vi "Main FPGA 5-axis Servo.vi"() -> ()   [LabVIEW 2014]
uses:
  <vilib>/Motion/MotorControl/_s/nism.encoder.config.ctl
  <vilib>/Motion/MotorControl/_s/nism.encoder.incremental.config.ctl
  <vilib>/Motion/MotorControl/_s/nism.incremental.indexCriteria.ctl
  <vilib>/Motion/MotorControl/_s/nism.pid.gains.fxp.18.ctl
  <vilib>/Motion/MotorControl/_s/nism.pi.v.outputRange.fxp.6.12.ctl
  <vilib>/Motion/MotorControl/_s/nism.mdo.splineData.ctl
  <vilib>/Motion/MotorControl/_s/nism.splineInterpolation.type.ctl
  <vilib>/Motion/SoftMotion/Synchronization/nism.softmotionScan.timerConfig.ctl
  <vilib>/Platform/TimedLoop/XDataNode/timing_clust.ctl
  <vilib>/Platform/TimedLoop/XDataNode/nitl_modes.ctl
  <vilib>/Platform/TimedLoop/XDataNode/wakeup.ctl
  <vilib>/Motion/MotorControl/_s/nism.digitalInputs.portA.ctl
  <vilib>/rvi/Emulation/niFpgaGetClockAttributes.vi
  <vilib>/rvi/Emulation/niFpgaSctlEmulationGetInTimedLoop.vi
  <vilib>/rvi/Emulation/niFpgaEmulationReportErrorSimple.vi
  Global FPGA 5-axis.vi
  <vilib>/Motion/MotorControl/_s/nism.interpretControlRegister.indexed.vi
  <vilib>/rvi/Emulation/niFpgaProcessEmulError.vi
  <vilib>/Motion/MotorControl/_s/nism.mdo.read.encoder.vi
  <vilib>/Motion/MotorControl/_s/nism.mdo.read.positionLoopSyncData.vi
  <vilib>/Motion/MotorControl/_s/nism.mdo.read.splineData.vi
  <vilib>/Motion/MotorControl/_s/nism.generateStatusRegister.indexed.vi
  <vilib>/rvi/eio/common/nirviEmuTemplateMethod_errors.vi
  <vilib>/rvi/Emulation/niFpgaCriticalErrorInLSC.vi
  <vilib>/Motion/MotorControl/_s/nism.splineInterpolation.fxp.3.index.vi
  <vilib>/Motion/MotorControl/_s/nism.pid.simple.fxp.index.2.vi
  <vilib>/Motion/MotorControl/_s/nism.mdo.handler.indexed.vi
  <vilib>/Motion/MotorControl/_s/nism.digitalFilter.indexed.vi
  <vilib>/Motion/MotorControl/_s/nism.interpretDIOControl.portA.multiple.vi
  <vilib>/Motion/MotorControl/_s/nism.generateDIOStatus.portA.indexed.2.vi
  <vilib>/Motion/SoftMotion/Synchronization/nism.rioScan.generateSyncScan.vi
  <vilib>/Motion/MotorControl/_s/nism.incremental.p.2.vi
  <vilib>/eio/EIONode/EIONode.xnode
  <vilib>/Platform/TimedLoop/XDataNode/XDataNode.xnode
  <vilib>/Motion/MotorControl/NI_SoftMotion_MotorControlIP.lvlib
  <vilib>/Platform/TimedLoop/XDataNode/XDNodeRunTimeDep.lvlib
  <vilib>/Motion/SoftMotion/Synchronization/NI_SoftMotion_Synchronization.lvlib
  <vilib>/rvi/Analysis/measure/butterworth/XNode/niFpgaButterworthFilter.xnode
panel:
  out "Interpolated Position":fxp<+/-,64,32>[](array[numeric])
  in  "Encoder Config (Manual)":T1={"active states"={"line a active high?"=FALSE, "line b active high?"=FALSE, "index active high?"=FALSE}, "index criteria"={"a"=FALSE, "b"=FALSE, "z"=FALSE}, "vel. filter coeffs."=[0, 0, 0]} caption="encoder config"
  in  "Velocity Filter Active?":bool
  in  "Reset Encoder 5":bool caption="reset"
  in  "Reset Encoder 4":bool caption="reset"
  in  "Reset Encoder 3":bool caption="reset"
  out "position loop sync":T4
  out "spline":T5 {"spline type" items=["cubic b spline", "catmull-rom spline", "linear"]}
  in  "Reset Encoder 2":bool caption="reset"
  out "Velocity Feedback":i16[](array[numeric])
  out "pos. error":i16[](array[numeric])
  out "pos. error exceeded":bool[](array[boolean])
  in  "calls per sample (vel)":u16=2000 caption="calls per sample"
  in  "Limit Ranges":T7[](array[typedef])=[{"output low"=0.0, "output high"=0.0}, {"output low"=0.0, "output high"=0.0}, {"output low"=0.0, "output high"=0.0}, {"output low"=0.0, "output high"=0.0}, {"output low"=0.0, "output high"=0.0}]
  in  "Gains":T8[](array[typedef])=[{"kp"=0.0, "kd"=0.0, "ki"=0.0}, {"kp"=0.0, "kd"=0.0, "ki"=0.0}, {"kp"=0.0, "kd"=0.0, "ki"=0.0}, {"kp"=0.0, "kd"=0.0, "ki"=0.0}, {"kp"=0.0, "kd"=0.0, "ki"=0.0}]
  out "AO Check":fxp<+/-,20,5>[](array[numeric])
  in  "AO Manual":fxp<+/-,20,5>[](array[numeric])=[0.0, 0.0, 0.0, 0.0, 0.0]
  out "Position Feedback":i32[](array[numeric])
  in  "Reset Encoder 1":bool caption="reset"
  out "corrected period":u16
  in  "AO Disabled?":bool
  out "PID loop time (ticks)":u32
  in  "AO Override?":bool
  in  "position error limit":i16=10000
  in  "Encoder filter value (us) Manual":u16=10
  out "encoder config":T1
  out "Home Limits":bool[](array[boolean])
  out "Fwd Limits":bool[](array[boolean])
  out "Rev Limits":bool[](array[boolean])
  out "Drive Enable":bool[](array[boolean])
  in  "Enable value":bool
  in  "Drive Enable override?":bool
  in  "Sync Value":bool
  in  "Sync Enable override?":bool
  out "Sync is Fault":bool
  out "Sync is Locked":bool
  # "Synchronization Loop"
  # "Control Status Loop"
  # "Notes: \n1. This VI provides the communication interface between the NI SoftMotion Engine and the LabVIEW FPGA Module. You must compile this VI for a specific FPGA target before use. After compiling, run the VI before running any of the Express VI examples. For information on moving this example to another FPGA target, refer to ni.com/info and enter info code fpgaex.\n\n2. Only use the Reset Axis button if you are unable to communicate with the axis by any other means. This button resets the device state machine and other VIs to a known state. After resetting the axis, switch the NI Scan Engine from Active Mode to Configuration Mode, then back to Active Mode, before attempting to enable the axis."
  # "(These two buttons \nare for testing\npurposes.)"
  # "(These two buttons \nare for testing\npurposes.)"
  # "Position/PID Loop"
  # "Parameter Check"
  # "AO Debug"
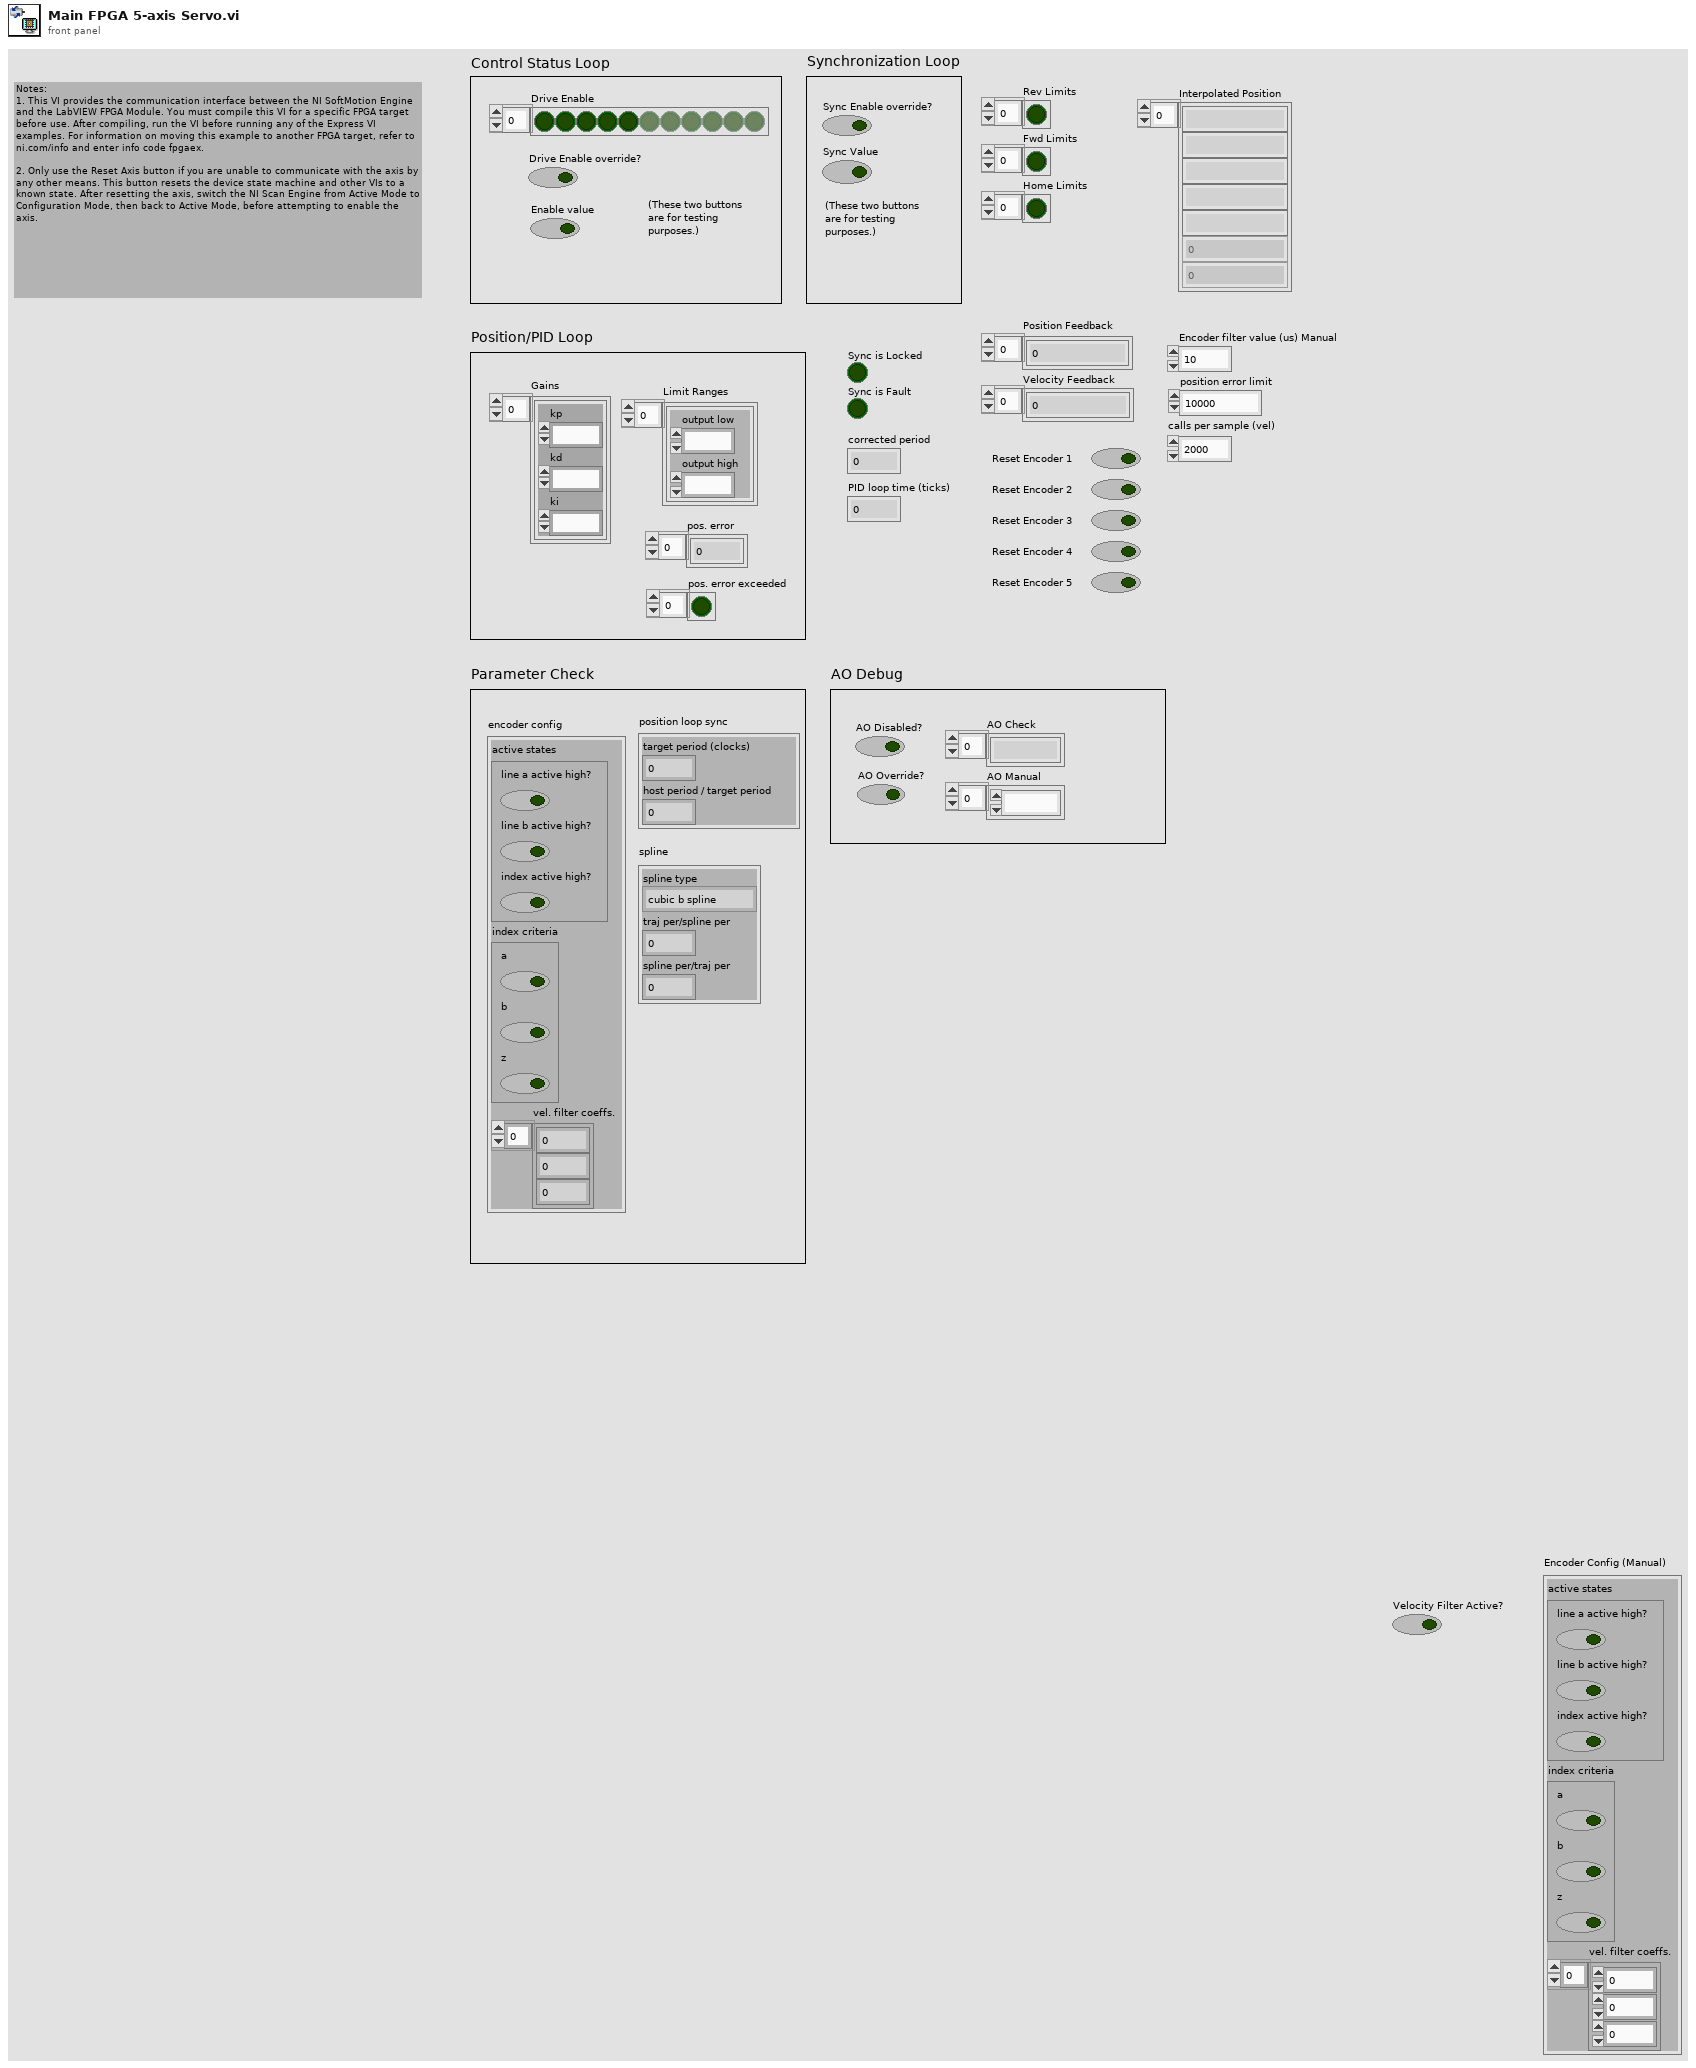
[diagram p1: front panel]
types:
  T1 = typedef "NI_SoftMotion_MotorControlIP.lvlib/nism.encoder.config.ctl" = cluster{"active states":T2, "index criteria":T3, "vel. filter coeffs.":i32[]}
  T2 = typedef "NI_SoftMotion_MotorControlIP.lvlib/nism.encoder.incremental.config.ctl" = cluster{"line a active high?":bool, "line b active high?":bool, "index active high?":bool}
  T3 = typedef "NI_SoftMotion_MotorControlIP.lvlib/nism.incremental.indexCriteria.ctl" = cluster{"a":bool, "b":bool, "z":bool}
  T4 = typedef "NI_SoftMotion_Synchronization.lvlib/nism.softmotionScan.timerConfig.ctl" = cluster{"target period (clocks)":u16, "host period / target period":u16}
  T5 = typedef "NI_SoftMotion_MotorControlIP.lvlib/nism.mdo.splineData.ctl" = cluster{"spline type":T6, "traj per/spline per":u16, "spline per/traj per":fxp<+,32,0>}
  T6 = typedef "NI_SoftMotion_MotorControlIP.lvlib/nism.splineInterpolation.type.ctl" = u16
  T7 = typedef "NI_SoftMotion_MotorControlIP.lvlib/nism.pi.v.outputRange.fxp.6.12.ctl" = cluster{"output low":fxp<+/-,18,6>, "output high":fxp<+/-,18,6>}
  T8 = typedef "NI_SoftMotion_MotorControlIP.lvlib/nism.pid.gains.fxp.18.ctl" = cluster{"kp":fxp<+,18,7>, "kd":fxp<+,18,7>, "ki":fxp<+,18,0>}
  T9 = typedef "XDNodeRunTimeDep.lvlib/timing_clust.ctl" = cluster{"Expected End [f-1]":u64, "Actual End [f-1]":u64, "Finished Late? [f-1]":bool, "Expected End [i-1]":u64, "Actual End [i-1]":u64, "Finished Late? [i-1]":bool, "Expected Start [i]":u64, "Actual Start [i]":u64, "Expected Start [f]":u64, "Actual Start [f]":u64, "Source Name":string, "Structure Name":string, "Period":i64, "Deadline":i64, "Offset":i64, "Start":i64, "Priority":i32, "Timeout":i32, "Mode":T10, "Wakeup Reason":T11, "Error":errorcluster, "Source Type":string, "Secondary Source Type":string, "Global End Time":u64, "Global Start Time":u64, "Frame Duration":u64, "Iteration Duration":u64, "Assigned CPU":i32, "I/O Scan Engine Mode":u32}
  T10 = typedef "XDNodeRunTimeDep.lvlib/nitl_modes.ctl" = enum32{"No Change", "Process missed periods, maintain original phase", "Discard missed periods, maintain original phase", "Process missed periods, ignore original phase", "Discard missed periods, ignore original phase"}
  T11 = typedef "XDNodeRunTimeDep.lvlib/wakeup.ctl" = enum32{"Normal", "Aborted", "Asynchronous wakeup", "Timing source error", "Timed loop error", "Timeout"}
  T12 = typedef "NI_SoftMotion_MotorControlIP.lvlib/nism.digitalInputs.portA.ctl" = cluster{"reverse limit":bool, "forward limit":bool, "home switch":bool, "digital input 0":bool, "digital input 1":bool, "digital input 2":bool, "digital input 3":bool}
  T13 = typedef "NI_SoftMotion_MotorControlIP.lvlib/nism.dio.portA.config.2.ctl" = cluster{"digital filter (us)":u16[], "safe state":T14[]}
  T14 = typedef "nism.safeStates.ctl" = enum8{"Low", "High", "No Change"}
  T15 = typedef "NI_SoftMotion_Synchronization.lvlib/nism.softmotionScan.timerControl.ctl" = cluster{"sm scan":bool, "sm scan count":u32, "sm scan enabled":bool}
  T16 = typedef "NI_SoftMotion_MotorControlIP.lvlib/nism.interpretControlRegister.stateTransition.ctl" = enum8{"Invalid", "Start --> Initializing", "Initializing --> Disabled", "Disabled --> Ready To Switch On", "Ready To Switch On --> Switched On", "Ready To Switch On --> Disable", "Switched On --> Operation Enable", "Switched On --> Ready To Switch On", "Switched On --> Disabled", "Operation Enable --> Switched On", "Operation Enable --> Ready To Switch On", "Operation Enable --> Disabled", "Fault --> Disabled", "Any --> Fault", "None"}
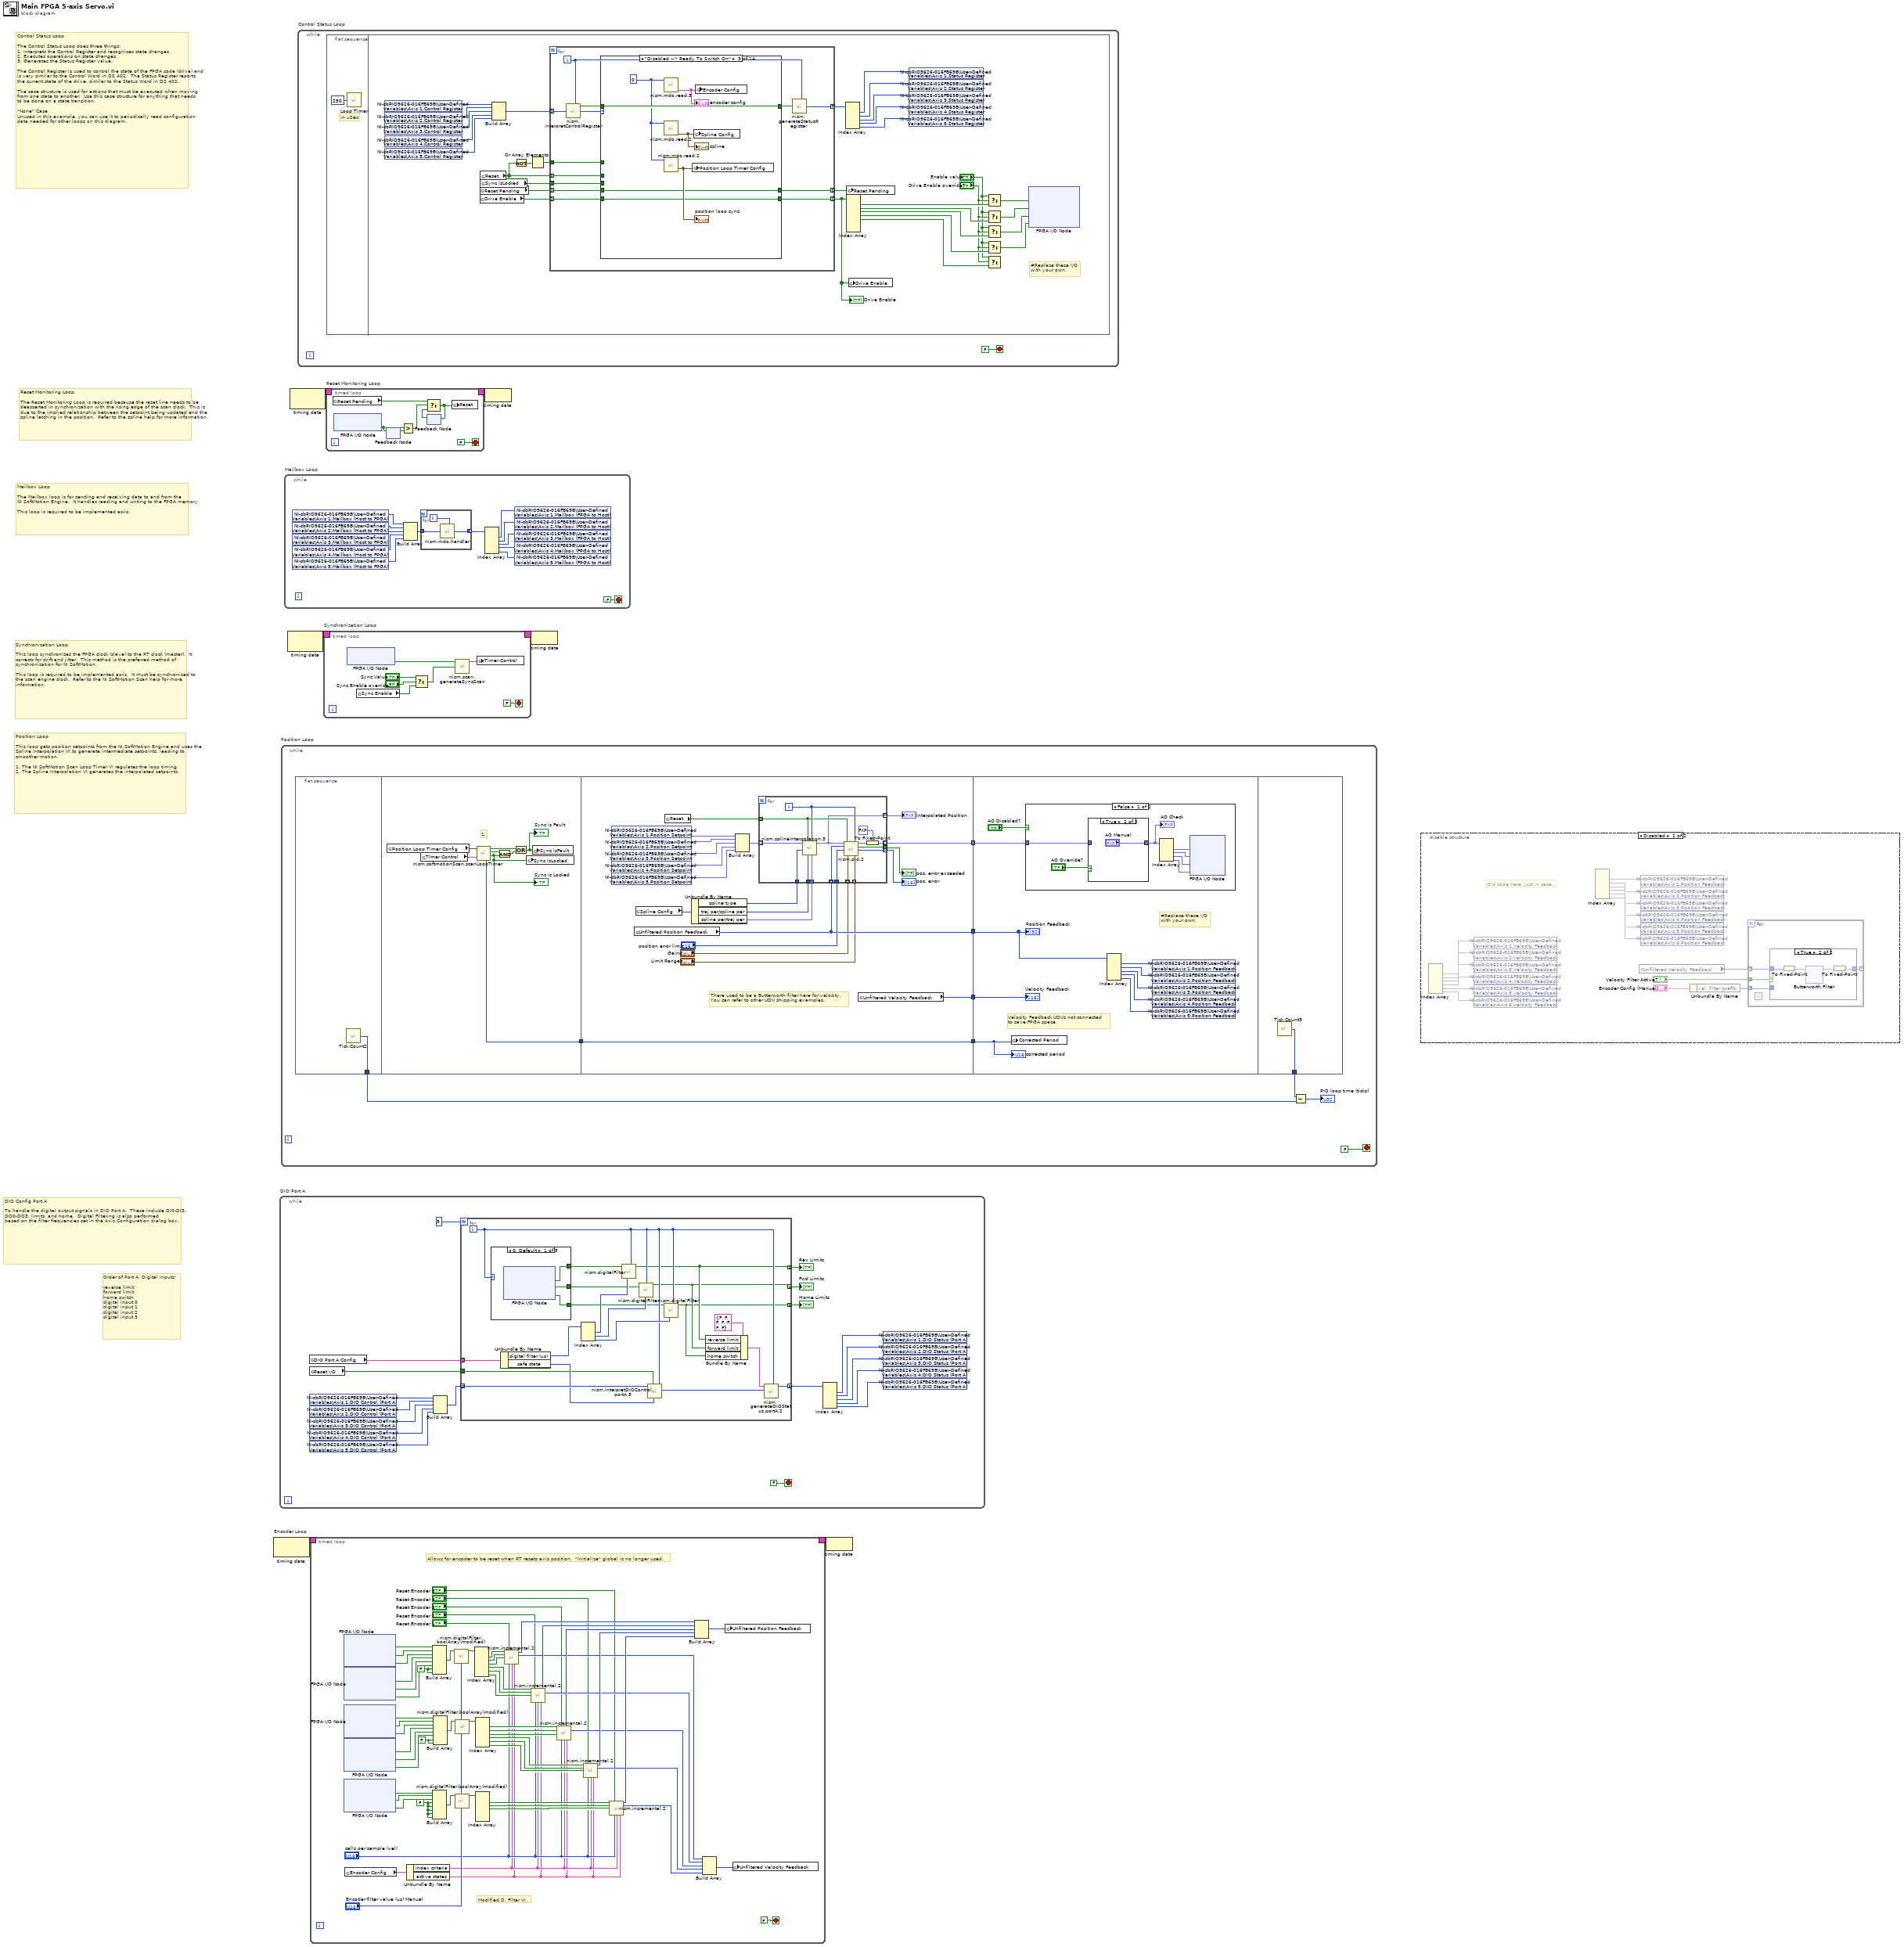
[diagram p0: block diagram]
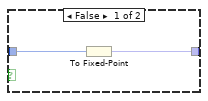
[diagram p2: hidden frame]
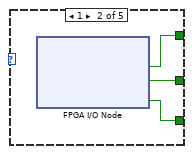
[diagram p4: hidden frame]
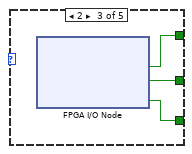
[diagram p5: hidden frame]
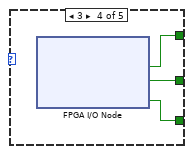
[diagram p6: hidden frame]
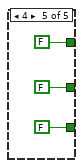
[diagram p7: hidden frame]
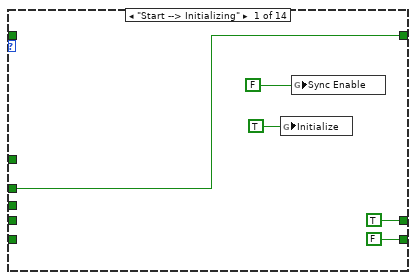
[diagram p10: hidden frame]
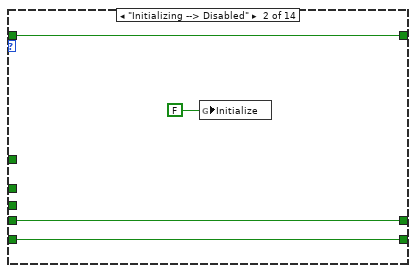
[diagram p11: hidden frame]
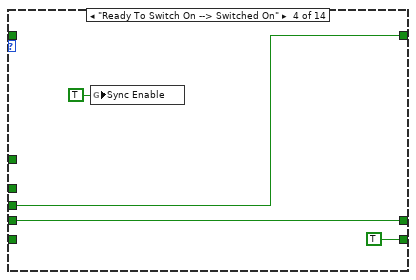
[diagram p12: hidden frame]
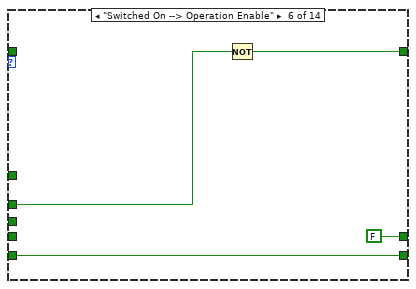
[diagram p14: hidden frame]
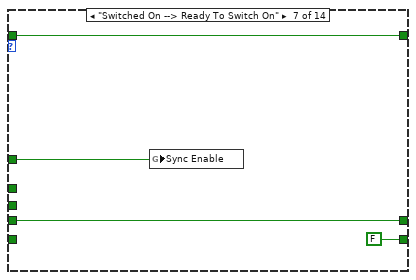
[diagram p15: hidden frame]
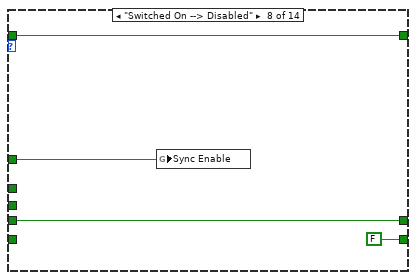
[diagram p16: hidden frame]
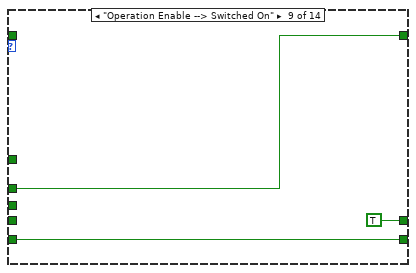
[diagram p17: hidden frame]
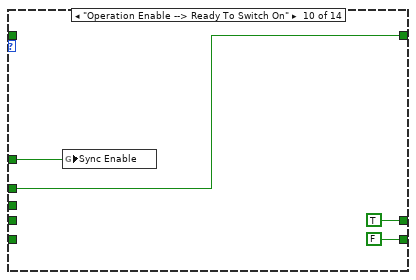
[diagram p18: hidden frame]
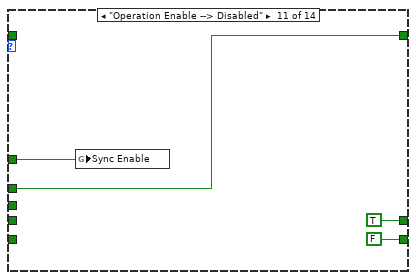
[diagram p19: hidden frame]
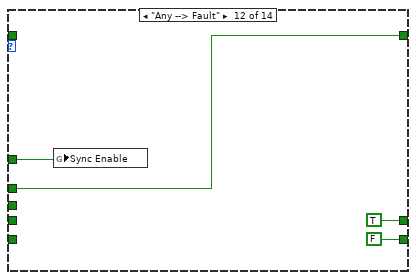
[diagram p20: hidden frame]
diagram:
  # "DIO Config Port A\n\nTo handle the digital output signals in DIO Port A.  These include DI0-DI3, DO0-DO3, limits, and home.  Digital Filtering is also performed\nbased on the filter frequencies set in the Axis Configuration dialog box."
  # "Order of Port A, Digital Inputs:\n\nreverse limit\nforward limit\nhome switch\ndigital input 0\ndigital input 1\ndigital input 2\ndigital input 3"
  # "Position Loop\n\nThis loop gets position setpoints from the NI SoftMotion Engine and uses the Spline Interpolation VI to generate intermediate setpoints, leading to smoother motion.\n\n1. The NI SoftMotion Scan Loop Timer VI regulates the loop timing. \n2. The Spline Interpolation VI generates the interpolated setpoints."
  # "Synchronization Loop\n\nThis loop synchronizes the FPGA clock (slave) to the RT clock (master).  It corrects for drift and jitter.  This method is the preferred method of synchronization for NI SoftMotion.\n\nThis loop is required to be implemented as-is.  It must be synchronized to the scan engine clock.  Refer to the NI SoftMotion Scan help for more information."
  # "Mailbox Loop\n\nThe Mailbox loop is for sending and receiving data to and from the \nNI SoftMotion Engine.  It handles reading and writing to the FPGA memory.\n\nThis loop is required to be implemented as-is."
  # "Reset Monitoring Loop\n\nThe Reset Monitoring Loop is required because the reset line needs to be deasserted in synchronization with the rising edge of the scan clock.  This is due to the implied relationship between the setpoint being updated and the spline latching in the position.  Refer to the spline help for more information."
  # "Control Status Loop\n\nThe Control Status Loop does three things:\n1. Interprets the Control Register and recognizes state changes.\n2. Executes operations on state changes.\n3. Generates the Status Register value.\n\nThe Control Register is used to control the state of the FPGA code (drive) and is very similar to the Control Word in DS 402.  The Status Register reports the current state of the drive, similar to the Status Word in DS 402.\n\nThe case structure is used for actions that must be executed when moving from one state to another.  Use this case structure for anything that needs to be done on a state transition.\n\n\"None\" Case\nUnused in this example, you can use it to periodically read configuration data needed for other loops on this diagram."
  n1 = node-c288() -> (w2:T9)  [unwired: 1 in]
  n2 = while "DIO Port A" {
    stop <- FALSE stop-if-true
    n3 = global read "Global FPGA 5-axis.vi" "DIO Port A Config"() -> (w24:T13)
    n4 = global read "Global FPGA 5-axis.vi" "Reset I/O"() -> (w23:bool)
    n5 = shared-variable "NI-sbRIO9626-016FB69B\\User-Defined Variables\\Axis 1.DIO Control (Port A)"() -> (w21:u32)  [unwired: 1 in, 1 out]
    n6 = shared-variable "NI-sbRIO9626-016FB69B\\User-Defined Variables\\Axis 2.DIO Control (Port A)"() -> (w20:u32)  [unwired: 1 in, 1 out]
    n7 = shared-variable "NI-sbRIO9626-016FB69B\\User-Defined Variables\\Axis 3.DIO Control (Port A)"() -> (w19:u32)  [unwired: 1 in, 1 out]
    n8 = shared-variable "NI-sbRIO9626-016FB69B\\User-Defined Variables\\Axis 4.DIO Control (Port A)"() -> (w18:u32)  [unwired: 1 in, 1 out]
    n9 = shared-variable "NI-sbRIO9626-016FB69B\\User-Defined Variables\\Axis 5.DIO Control (Port A)"() -> (w17:u32)  [unwired: 1 in, 1 out]
    n10 = Build Array(w21, w20, w19, w18, w17) -> (w16:u32[])
    n11 = for {
      N: 5 -> [_]
      tunnel: [w43] -> w10 mode=indexing
      tunnel: w16 -> [w42] mode=indexing
      tunnel: w24 -> [w39]
      tunnel: w23 -> [w37]
      tunnel: [w28] -> w9 mode=indexing
      tunnel: [w27] -> w8 mode=indexing
      tunnel: [w26] -> w7 mode=indexing
      i -> [w32]
      n12 = case shown="0, Default" w32 {
        tunnel: [w47 w50 w53 w56 FALSE ("RMC/DIO44")] -> w31
        tunnel: [w45 w48 w51 w54 FALSE ("RMC/DIO61")] -> w30
        tunnel: [w46 w49 w52 w55 FALSE ("RMC/DIO77")] -> w29
        frame 0, Default {
          n13 = xnode "FPGA I/O Node"() -> ("RMC/DIO29"=w47:bool, "RMC/DIO93"=w46:bool, "RMC/DIO11"=w45:bool)  [unwired: 3 in, 3 out]
        }
        frame 1 {
          n14 = xnode "FPGA I/O Node"() -> ("RMC/DIO44"=w50:bool, "RMC/DIO77"=w49:bool, "RMC/DIO61"=w48:bool)  [unwired: 3 in, 3 out]
        }
        frame 2 {
          n15 = xnode "FPGA I/O Node"() -> ("RMC/DIO31"=w53:bool, "RMC/DIO95"=w52:bool, "RMC/DIO13"=w51:bool)  [unwired: 3 in, 3 out]
        }
        frame 3 {
          n16 = xnode "FPGA I/O Node"() -> ("RMC/DIO47"=w56:bool, "RMC/DIO46"=w55:bool, "RMC/DIO79"=w54:bool)  [unwired: 3 in, 3 out]
        }
        frame 4 {
        }
      }
      n17 = Unbundle By Name(w39) -> ("digital filter (us)"=w33:u16[], "safe state"=w38:T14[])
      n18 = Index Array(array=w33) -> (element #1=w34:u16, element #2=w35:u16, element #3=w36:u16)  [unwired: 3 in]
      n19 = call-poly <vilib>:"nism.digitalFilter.vi"("index"=w32, "filter value (us)"=w34, "input signal"=w31) -> ("output signal"=w28:bool)  [unwired: 8 in]
      n20 = call-poly <vilib>:"nism.digitalFilter.vi"("index"=w32, "filter value (us)"=w35, "input signal"=w29) -> ("output signal"=w27:bool)  [unwired: 8 in]
      n21 = call-poly <vilib>:"nism.interpretDIOControl.portA.3.vi"("index"=w32, "safe state"=w38, "reset"=w37, "dio control(port a)"=w42) -> ("reset latches"=w44:u8)  [unwired: 6 in, 1 out]
      n22 = call-poly <vilib>:"nism.digitalFilter.vi"("index"=w32, "filter value (us)"=w36, "input signal"=w30) -> ("output signal"=w26:bool)  [unwired: 8 in]
      n23 = Bundle By Name(cluster=T12 {"reverse limit"=FALSE, "forward limit"=FALSE, "home switch"=FALSE, "digital input 0"=FALSE, "digital input 1"=FALSE, "digital input 2"=FALSE, "digital input 3"=FALSE} ("$(driveInterface.digitalInputs.shortName)"), "reverse limit"=w28, "forward limit"=w27, "home switch"=w26) -> (w40:T12)
      n24 = call-poly <vilib>:"nism.generateDIOStatus.portA.2.vi"("index"=w32, "reset latches"=w44, "digital inputs"=w40) -> ("dio status(port a)"=w43:u32)  [unwired: 8 in]
    }
    "Rev Limits" <- w9
    "Fwd Limits" <- w8
    "Home Limits" <- w7
    n25 = Index Array(array=w10) -> (element #1=w15:u32, element #2=w14:u32, element #3=w13:u32, element #4=w12:u32, element #5=w11:u32)  [unwired: 5 in]
    n26 = shared-variable "NI-sbRIO9626-016FB69B\\User-Defined Variables\\Axis 1.DIO Status (Port A)"(w15) -> ()  [unwired: 1 in, 1 out]
    n27 = shared-variable "NI-sbRIO9626-016FB69B\\User-Defined Variables\\Axis 2.DIO Status (Port A)"(w14) -> ()  [unwired: 1 in, 1 out]
    n28 = shared-variable "NI-sbRIO9626-016FB69B\\User-Defined Variables\\Axis 3.DIO Status (Port A)"(w13) -> ()  [unwired: 1 in, 1 out]
    n29 = shared-variable "NI-sbRIO9626-016FB69B\\User-Defined Variables\\Axis 4.DIO Status (Port A)"(w12) -> ()  [unwired: 1 in, 1 out]
    n30 = shared-variable "NI-sbRIO9626-016FB69B\\User-Defined Variables\\Axis 5.DIO Status (Port A)"(w11) -> ()  [unwired: 1 in, 1 out]
  }
  n31 = while "Position Loop" {
    stop <- FALSE stop-if-true
    n32 = flat-sequence {
      tunnel: [w69] -> w63
      tunnel: [w70] -> w66
      tunnel: [w94] -> w67
      tunnel: w66 -> [w94]
      tunnel: [w84] -> w65
      tunnel: [w88] -> w61
      tunnel: [w79] -> w60
      tunnel: w67 -> [w124]
      tunnel: w65 -> [w115]
      tunnel: w61 -> [w123]
      tunnel: w60 -> [w121]
      tunnel: [w134] -> w64
      frame #0 {
        n33 = call "Tick Count2"() -> ("Tick Count(Ticks)"=w69:u32)
      }
      frame #1 {
        # "1."
        n34 = global read "Global FPGA 5-axis.vi" "Position Loop Timer Config"() -> (w72:T4)
        n35 = global read "Global FPGA 5-axis.vi" "Timer Control"() -> (w71:T15)
        n36 = call <vilib>:"nism.softmotionScan.scanLoopTimer.vi"("timer control"=w71, "timer config"=w72) -> ("scan running?"=w74:bool, "finished late?"=w76:bool, "fault occurred?"=w77:bool, "corrected period"=w70:u16)  [unwired: 5 in, 1 out]
        "Sync is Locked" <- w74
        n37 = Compound Arithmetic op=AND(w76, w74) -> (w75:bool)
        n38 = Compound Arithmetic op=OR(w77, w75) -> (w73:bool)
        "Sync is Fault" <- w73
        n39 = global write "Global FPGA 5-axis.vi" "Sync isLocked"(w74) -> ()
        n40 = global write "Global FPGA 5-axis.vi" "Sync isFault"(w73) -> ()
      }
      frame #2 {
        # "There used to be a Butterworth filter here for velocity.  \nYou can refer to other UDV shipping examples."
        n41 = shared-variable "NI-sbRIO9626-016FB69B\\User-Defined Variables\\Axis 1.Position Setpoint"() -> (w89:fxp<+/-,64,32>)  [unwired: 1 in, 1 out]
        n42 = shared-variable "NI-sbRIO9626-016FB69B\\User-Defined Variables\\Axis 2.Position Setpoint"() -> (w93:fxp<+/-,64,32>)  [unwired: 1 in, 1 out]
        n43 = shared-variable "NI-sbRIO9626-016FB69B\\User-Defined Variables\\Axis 3.Position Setpoint"() -> (w92:fxp<+/-,64,32>)  [unwired: 1 in, 1 out]
        n44 = shared-variable "NI-sbRIO9626-016FB69B\\User-Defined Variables\\Axis 4.Position Setpoint"() -> (w91:fxp<+/-,64,32>)  [unwired: 1 in, 1 out]
        n45 = shared-variable "NI-sbRIO9626-016FB69B\\User-Defined Variables\\Axis 5.Position Setpoint"() -> (w90:fxp<+/-,64,32>)  [unwired: 1 in, 1 out]
        n46 = global read "Global FPGA 5-axis.vi" "Unfiltered Position Feedback"() -> (w84:i32[])
        n47 = global read "Global FPGA 5-axis.vi" "Spline Config"() -> (w95:T5)
        n48 = global read "Global FPGA 5-axis.vi" "Reset"() -> (w86:bool[])
        n49 = Unbundle By Name(w95) -> ("spline type"=w98:T6, "traj per/spline per"=w97:u16, "spline per/traj per"=w96:fxp<+,32,0>)
        n50 = Build Array(w89, w93, w92, w91, w90) -> (w87:fxp<+/-,64,32>[])
        n51 = for {
          tunnel: w98 -> [w114]
          tunnel: w97 -> [w113]
          tunnel: w96 -> [w112]
          tunnel: "Limit Ranges" -> [w111] mode=indexing
          tunnel: [w101] -> w88 mode=indexing
          tunnel: w87 -> [w110] mode=indexing
          tunnel: w86 -> [w108] mode=indexing
          tunnel: w84 -> [w107] mode=indexing
          tunnel: "position error limit" -> [w106]
          tunnel: [w105] -> w81 mode=indexing
          tunnel: [w104] -> w80 mode=indexing
          tunnel: "Gains" -> [w100] mode=indexing
          tunnel: [w99] -> w78 mode=indexing
          i -> [w109]
          n52 = call-poly <vilib>:"nism.splineInterpolation.3.vi"("1 / calls per sample"=w112, "index"=w109, "calls per sample"=w113, "reset"=w108, "spline type"=w114, "x"=w110) -> ("xi"=w99:fxp<+/-,64,32>)  [unwired: 4 in, 1 out]
          n53 = call-poly <vilib>:"nism.pid.2.vi"("position setpoint"=w99, "position feedback"=w107, "position error limit"=w106, "reset"=w108, "gains"=w100, "index"=w109, "output range"=w111) -> ("current setpoint"=w102:fxp<+/-,18,6>, "pos. error exceeded"=w105:bool, "position error"=w104:i16)  [unwired: 10 in]
          n54 = To Fixed-Point(fixed-point type=fxp<+/-,20,5> 0.0 ("AO 1"), number=w102) -> (fixed-point=w101:fxp<+/-,20,5>)
        }
        "pos. error exceeded" <- w81
        "pos. error" <- w80
        "Interpolated Position" <- w78
        n55 = global read "Global FPGA 5-axis.vi" "Unfiltered Velocity Feedback"() -> (w79:i16[])
      }
      frame #3 {
        # "Velocity Feedback UDVs not connected\nto save FPGA space."
        # "#Replace these I/O\nwith your own."
        n56 = global write "Global FPGA 5-axis.vi" "Corrected Period"(w124) -> ()
        n57 = case shown="False" "AO Disabled?" {
          tunnel: w123 -> [w130 _]
          frame False {
            n58 = case shown="True" "AO Override?" {
              tunnel: w130 -> [w132 _]
              tunnel: [w132 "AO Manual"] -> w129
              frame False {
              }
              frame True {
              }
            }
            "AO Check" <- w129
            n59 = Index Array(array=w129) -> (element #1=w128:fxp<+/-,20,5>, element #2=w127:fxp<+/-,20,5>, element #3=w126:fxp<+/-,20,5>, element #4=w125:fxp<+/-,20,5>)  [unwired: 4 in]
            n60 = xnode "FPGA I/O Node"("AO0"=w128, "AO1"=w127, "AO2"=w126, "AO3"=w125) -> ()  [unwired: 4 in, 4 out]
          }
          frame True {
          }
        }
        n61 = Index Array(array=w115) -> (element #1=w120:i32, element #2=w119:i32, element #3=w118:i32, element #4=w117:i32, element #5=w116:i32)  [unwired: 5 in]
        n62 = shared-variable "NI-sbRIO9626-016FB69B\\User-Defined Variables\\Axis 1.Position Feedback"(w120) -> ()  [unwired: 1 in, 1 out]
        n63 = shared-variable "NI-sbRIO9626-016FB69B\\User-Defined Variables\\Axis 2.Position Feedback"(w119) -> ()  [unwired: 1 in, 1 out]
        n64 = shared-variable "NI-sbRIO9626-016FB69B\\User-Defined Variables\\Axis 3.Position Feedback"(w118) -> ()  [unwired: 1 in, 1 out]
        n65 = shared-variable "NI-sbRIO9626-016FB69B\\User-Defined Variables\\Axis 4.Position Feedback"(w117) -> ()  [unwired: 1 in, 1 out]
        n66 = shared-variable "NI-sbRIO9626-016FB69B\\User-Defined Variables\\Axis 5.Position Feedback"(w116) -> ()  [unwired: 1 in, 1 out]
        "corrected period" <- w124
        "Position Feedback" <- w115
        "Velocity Feedback" <- w121
      }
      frame #4 {
        n67 = call "Tick Count3"() -> ("Tick Count(Ticks)"=w134:u32)
      }
    }
    n68 = Subtract(x=w64, y=w63) -> (x-y=→"PID loop time (ticks)":u32)
  }
  n69 = while "Mailbox Loop" {
    stop <- FALSE stop-if-true
    n70 = shared-variable "NI-sbRIO9626-016FB69B\\User-Defined Variables\\Axis 1.Mailbox (Host to FPGA)"() -> (w144:u64)  [unwired: 1 in, 1 out]
    n71 = shared-variable "NI-sbRIO9626-016FB69B\\User-Defined Variables\\Axis 2.Mailbox (Host to FPGA)"() -> (w143:u64)  [unwired: 1 in, 1 out]
    n72 = shared-variable "NI-sbRIO9626-016FB69B\\User-Defined Variables\\Axis 3.Mailbox (Host to FPGA)"() -> (w142:u64)  [unwired: 1 in, 1 out]
    n73 = shared-variable "NI-sbRIO9626-016FB69B\\User-Defined Variables\\Axis 4.Mailbox (Host to FPGA)"() -> (w141:u64)  [unwired: 1 in, 1 out]
    n74 = shared-variable "NI-sbRIO9626-016FB69B\\User-Defined Variables\\Axis 5.Mailbox (Host to FPGA)"() -> (w140:u64)  [unwired: 1 in, 1 out]
    n75 = Build Array(w144, w143, w142, w141, w140) -> (w146:u64[])
    n76 = for {
      tunnel: w146 -> [w150] mode=indexing
      tunnel: [w149] -> w145 mode=indexing
      i -> [w148]
      n77 = call-poly <vilib>:"nism.mdo.handler.vi"("mbox (host to fpga)"=w150, "axis index"=w148) -> ("mbox (fpga to host)"=w149:u64)  [unwired: 7 in]
    }
    n78 = Index Array(array=w145) -> (element #1=w139:u64, element #2=w138:u64, element #3=w137:u64, element #4=w136:u64, element #5=w135:u64)  [unwired: 5 in]
    n79 = shared-variable "NI-sbRIO9626-016FB69B\\User-Defined Variables\\Axis 1.Mailbox (FPGA to Host)"(w139) -> ()  [unwired: 1 in, 1 out]
    n80 = shared-variable "NI-sbRIO9626-016FB69B\\User-Defined Variables\\Axis 2.Mailbox (FPGA to Host)"(w138) -> ()  [unwired: 1 in, 1 out]
    n81 = shared-variable "NI-sbRIO9626-016FB69B\\User-Defined Variables\\Axis 3.Mailbox (FPGA to Host)"(w137) -> ()  [unwired: 1 in, 1 out]
    n82 = shared-variable "NI-sbRIO9626-016FB69B\\User-Defined Variables\\Axis 4.Mailbox (FPGA to Host)"(w136) -> ()  [unwired: 1 in, 1 out]
    n83 = shared-variable "NI-sbRIO9626-016FB69B\\User-Defined Variables\\Axis 5.Mailbox (FPGA to Host)"(w135) -> ()  [unwired: 1 in, 1 out]
  }
  n84 = node-c288() -> (w6:T9)  [unwired: 1 in]
  n85 = node-c288() -> (w4:T9)  [unwired: 1 in]
  n86 = while "Control Status Loop" {
    stop <- FALSE stop-if-true
    n87 = flat-sequence {
      frame #0 {
        # "in uSec"
        n88 = call "Loop Timer"("Count(uSec)"=u32 250) -> ()  [unwired: 1 out]
      }
      frame #1 {
        # "#Replace these I/O\nwith your own."
        n89 = shared-variable "NI-sbRIO9626-016FB69B\\User-Defined Variables\\Axis 1.Control Register"() -> (w173:u32)  [unwired: 1 in, 1 out]
        n90 = shared-variable "NI-sbRIO9626-016FB69B\\User-Defined Variables\\Axis 2.Control Register"() -> (w172:u32)  [unwired: 1 in, 1 out]
        n91 = shared-variable "NI-sbRIO9626-016FB69B\\User-Defined Variables\\Axis 3.Control Register"() -> (w171:u32)  [unwired: 1 in, 1 out]
        n92 = shared-variable "NI-sbRIO9626-016FB69B\\User-Defined Variables\\Axis 4.Control Register"() -> (w170:u32)  [unwired: 1 in, 1 out]
        n93 = shared-variable "NI-sbRIO9626-016FB69B\\User-Defined Variables\\Axis 5.Control Register"() -> (w169:u32)  [unwired: 1 in, 1 out]
        n94 = global read "Global FPGA 5-axis.vi" "Reset Pending"() -> (w177:bool[])
        n95 = global read "Global FPGA 5-axis.vi" "Drive Enable"() -> (w176:bool[])
        n96 = global read "Global FPGA 5-axis.vi" "Reset"() -> (w178:bool[])
        n97 = global read "Global FPGA 5-axis.vi" "Sync isLocked"() -> (w183:bool)
        n98 = Build Array(w173, w172, w171, w170, w169) -> (w182:u32[])
        n99 = Not(x=w178) -> (.not. x?=w180:bool[])
        n100 = Or Array Elements(Boolean array=w180) -> (logical OR=w179:bool)
        n101 = for {
          tunnel: w178 -> [w192] mode=indexing
          tunnel: w183 -> [w191]
          tunnel: w182 -> [w193] mode=indexing
          tunnel: [w190] -> w174 mode=indexing
          tunnel: [w189] -> w181 mode=indexing
          tunnel: [w188] -> w175 mode=indexing
          tunnel: w179 -> [w187]
          tunnel: w177 -> [w186] mode=indexing
          tunnel: w176 -> [w185] mode=indexing
          i -> [w194]
          n102 = call-poly <vilib>:"nism.interpretControlRegister.vi"("control register"=w193, "axis index"=w194) -> ("transition occurred"=w195:bool, "state transition"=w184:T16)  [unwired: 6 in]
          n103 = case shown="\"Disabled --> Ready To Switch On\"" w184 {
            tunnel: w195 -> [_ w205 w212 _ w219 _ w227 w231 _ _ _ _ w251 _]
            tunnel: [w201 w205 w212 w214 w219 w223 w227 w231 w233 w236 w240 w244 w250 _] -> w196
            tunnel: w192 -> [w201 _ _ _ _ w222 _ _ w233 w236 w240 w244 _ _]
            tunnel: w191 -> [_ _ _ w214 _ _ _ _ _ _ _ _ _ _]
            tunnel: [TRUE ("Write.Reset Pending") w204 w209 w213 w218 FALSE ("Write.Reset Pending") w224 w228 TRUE ("Write.Reset Pending") TRUE ("Write.Reset Pending") TRUE ("Write.Reset Pending") TRUE ("Write.Reset Pending") w248 w253] -> w189
            tunnel: [FALSE ("Write.Drive Enable") w203 w208 TRUE ("Write.Drive Enable") w217 w220 FALSE ("Write.Drive Enable") FALSE ("Write.Drive Enable") w232 FALSE ("Write.Drive Enable") FALSE ("Write.Drive Enable") FALSE ("Write.Drive Enable") w247 w252] -> w188
            tunnel: w187 -> [_ _ _ _ _ _ w225 w229 _ w235 w239 w243 w249 _]
            tunnel: w186 -> [_ w204 w209 w213 w218 _ w224 w228 _ _ _ _ w248 w253]
            tunnel: w185 -> [_ w203 w208 _ w217 w220 _ _ w232 _ _ _ w247 w252]
            frame "Start --> Initializing" {
              n104 = global write "Global FPGA 5-axis.vi" "Initialize"(TRUE ("Initialize")) -> ()
              n105 = global write "Global FPGA 5-axis.vi" "Sync Enable"(FALSE ("Sync Enable")) -> ()
            }
            frame "Initializing --> Disabled" {
              n106 = global write "Global FPGA 5-axis.vi" "Initialize"(FALSE ("Initialize")) -> ()
            }
            frame "Disabled --> Ready To Switch On" {
              w206 = 0 ("axis index")
              n107 = call-poly <vilib>:"nism.mdo.read.3.vi"("axis index"=w206) -> ("encoder config"=w207:T1)  [unwired: 10 in]
              "encoder config" <- w207
              n108 = call-poly <vilib>:"nism.mdo.read.2.vi"("axis index"=w206) -> ("spline"=w211:T5)  [unwired: 10 in]
              "spline" <- w211
              n109 = call-poly <vilib>:"nism.mdo.read.2.vi"("axis index"=w206) -> ("position loop sync"=w210:T4)  [unwired: 10 in]
              "position loop sync" <- w210
              n110 = global write "Global FPGA 5-axis.vi" "Position Loop Timer Config"(w210) -> ()
              n111 = global write "Global FPGA 5-axis.vi" "Spline Config"(w211) -> ()
              n112 = global write "Global FPGA 5-axis.vi" "Encoder Config"(w207) -> ()
            }
            frame "Ready To Switch On --> Switched On" {
              n113 = global write "Global FPGA 5-axis.vi" "Sync Enable"(TRUE ("Sync Enable")) -> ()
            }
            frame "Ready To Switch On --> Disable" {
            }
            frame "Switched On --> Operation Enable" {
              n114 = Not(x=w222) -> (.not. x?=w223:bool)
            }
            frame "Switched On --> Ready To Switch On" {
              n115 = global write "Global FPGA 5-axis.vi" "Sync Enable"(w225) -> ()
            }
            frame "Switched On --> Disabled" {
              n116 = global write "Global FPGA 5-axis.vi" "Sync Enable"(w229) -> ()
            }
            frame "Operation Enable --> Switched On" {
            }
            frame "Operation Enable --> Ready To Switch On" {
              n117 = global write "Global FPGA 5-axis.vi" "Sync Enable"(w235) -> ()
            }
            frame "Operation Enable --> Disabled" {
              n118 = global write "Global FPGA 5-axis.vi" "Sync Enable"(w239) -> ()
            }
            frame "Any --> Fault" {
              n119 = global write "Global FPGA 5-axis.vi" "Sync Enable"(w243) -> ()
            }
            frame "Fault --> Disabled" {
              # "wait one cycle for clear faults to have taken effect"
              n120 = global write "Global FPGA 5-axis.vi" "Sync Enable"(w249) -> ()
              n121 = Not(x=w251) -> (.not. x?=w250:bool)
            }
            frame "None", Default {
            }
          }
          n122 = call-poly <vilib>:"nism.generateStatusRegister.vi"("transition success"=w196, "axis index"=w194) -> ("status register"=w190:u32)  [unwired: 7 in]
        }
        "Drive Enable" <- w175
        n123 = Index Array(array=w174) -> (element #1=w168:u32, element #2=w167:u32, element #3=w166:u32, element #4=w165:u32, element #5=w164:u32)  [unwired: 5 in]
        n124 = global write "Global FPGA 5-axis.vi" "Reset Pending"(w181) -> ()
        n125 = Index Array(array=w175) -> (element #1=w163:bool, element #2=w162:bool, element #3=w161:bool, element #4=w160:bool, element #5=w159:bool)  [unwired: 8 in, 3 out]
        n126 = global write "Global FPGA 5-axis.vi" "Drive Enable"(w175) -> ()
        n127 = shared-variable "NI-sbRIO9626-016FB69B\\User-Defined Variables\\Axis 1.Status Register"(w168) -> ()  [unwired: 1 in, 1 out]
        n128 = shared-variable "NI-sbRIO9626-016FB69B\\User-Defined Variables\\Axis 2.Status Register"(w167) -> ()  [unwired: 1 in, 1 out]
        n129 = shared-variable "NI-sbRIO9626-016FB69B\\User-Defined Variables\\Axis 3.Status Register"(w166) -> ()  [unwired: 1 in, 1 out]
        n130 = shared-variable "NI-sbRIO9626-016FB69B\\User-Defined Variables\\Axis 4.Status Register"(w165) -> ()  [unwired: 1 in, 1 out]
        n131 = shared-variable "NI-sbRIO9626-016FB69B\\User-Defined Variables\\Axis 5.Status Register"(w164) -> ()  [unwired: 1 in, 1 out]
        n132 = Select(t="Enable value", s="Drive Enable override?", f=w163) -> (s? t:f=w158:bool)
        n133 = Select(t="Enable value", s="Drive Enable override?", f=w162) -> (s? t:f=w157:bool)
        n134 = Select(t="Enable value", s="Drive Enable override?", f=w161) -> (s? t:f=w156:bool)
        n135 = Select(t="Enable value", s="Drive Enable override?", f=w160) -> (s? t:f=w155:bool)
        n136 = Select(t="Enable value", s="Drive Enable override?", f=w159) -> ()  [unwired: 1 out]
        n137 = xnode "FPGA I/O Node"("RMC/DIO28"=w158, "RMC/DIO12"=w157, "RMC/DIO30"=w156, "RMC/DIO14"=w155) -> ()  [unwired: 4 in, 4 out]
      }
    }
  }
  n138 = timed-loop "Encoder Loop" {
    timing: w2 -> [_]
    timing-out: [_] -> w1
    stop <- FALSE stop-if-true
    w254 = FALSE ("element")
    w273 = FALSE ("element")
    w289 = FALSE ("element")
    # "Allows for encoder to be reset when RT resets axis position.  \"Initialize\" global is no longer used."
    # "Modified D. Filter VI."
    n139 = xnode "FPGA I/O Node"() -> ("RMC/DIO60"=w313:bool, "RMC/DIO42"=w314:bool, "RMC/DIO75"=w312:bool)  [unwired: 3 in, 3 out]
    n140 = xnode "FPGA I/O Node"() -> ("RMC/DIO59"=w294:bool, "RMC/DIO92"=w293:bool, "RMC/DIO10"=w292:bool)  [unwired: 3 in, 3 out]
    n141 = xnode "FPGA I/O Node"() -> ("RMC/DIO74"=w285:bool, "RMC/DIO27"=w284:bool, "RMC/DIO91"=w283:bool)  [unwired: 3 in, 3 out]
    n142 = xnode "FPGA I/O Node"() -> ("RMC/DIO9"=w282:bool, "RMC/DIO41"=w281:bool, "RMC/DIO26"=w280:bool)  [unwired: 3 in, 3 out]
    n143 = xnode "FPGA I/O Node"() -> ("RMC/DIO58"=w270:bool, "RMC/DIO40"=w271:bool, "RMC/DIO73"=w272:bool)  [unwired: 3 in, 3 out]
    n144 = global read "Global FPGA 5-axis.vi" "Encoder Config"() -> (w258:T1)
    n145 = Unbundle By Name(w258) -> ("index criteria"=w261:T3, "active states"=w260:T2)
    n146 = Build Array(w313, w314, w312, w294, w293, w292, w289, w289) -> (w311:bool[])
    n147 = Build Array(w270, w271, w272, w254, w254, w254, w254, w254) -> (w269:bool[])
    n148 = Build Array(w285, w284, w283, w282, w281, w280, w273, w273) -> (w290:bool[])
    n149 = call "nism.digitalFilter.boolArray(modified).vi"("filter value (us)"="Encoder filter value (us) Manual", "input signal"=w311) -> ("output signal"=w310:bool[])  [unwired: 9 in]
    n150 = call "nism.digitalFilter.boolArray(modified).vi"("filter value (us)"="Encoder filter value (us) Manual", "input signal"=w269) -> ("output signal"=w268:bool[])  [unwired: 9 in]
    n151 = call "nism.digitalFilter.boolArray(modified).vi"("filter value (us)"="Encoder filter value (us) Manual", "input signal"=w290) -> ("output signal"=w291:bool[])  [unwired: 9 in]
    n152 = Index Array(array=w310) -> (element #1=w309:bool, element #2=w308:bool, element #3=w307:bool, element #4=w288:bool, element #5=w287:bool, element #6=w286:bool)  [unwired: 6 in]
    n153 = Index Array(array=w268) -> (element #1=w267:bool, element #2=w266:bool, element #3=w265:bool)  [unwired: 6 in, 3 out]
    n154 = Index Array(array=w291) -> (element #1=w279:bool, element #2=w278:bool, element #3=w277:bool, element #4=w276:bool, element #5=w275:bool, element #6=w274:bool)  [unwired: 6 in]
    n155 = call-poly <vilib>:"nism.incremental.2.vi"("a phase"=w309, "reset"="Reset Encoder 1", "b phase"=w308, "z phase"=w307, "calls per sample"="calls per sample (vel)", "index criteria"=w261, "active states"=w260) -> ("encoder position"=w306:i32, "velocity"=w299:i16)  [unwired: 5 in, 2 out]
    n156 = call-poly <vilib>:"nism.incremental.2.vi"("a phase"=w288, "reset"="Reset Encoder 2", "b phase"=w287, "z phase"=w286, "calls per sample"="calls per sample (vel)", "index criteria"=w261, "active states"=w260) -> ("encoder position"=w305:i32, "velocity"=w298:i16)  [unwired: 5 in, 2 out]
    n157 = call-poly <vilib>:"nism.incremental.2.vi"("a phase"=w279, "reset"="Reset Encoder 3", "b phase"=w278, "z phase"=w277, "calls per sample"="calls per sample (vel)", "index criteria"=w261, "active states"=w260) -> ("encoder position"=w304:i32, "velocity"=w297:i16)  [unwired: 5 in, 2 out]
    n158 = call-poly <vilib>:"nism.incremental.2.vi"("a phase"=w276, "reset"="Reset Encoder 4", "b phase"=w275, "z phase"=w274, "calls per sample"="calls per sample (vel)", "index criteria"=w261, "active states"=w260) -> ("encoder position"=w303:i32, "velocity"=w296:i16)  [unwired: 5 in, 2 out]
    n159 = call-poly <vilib>:"nism.incremental.2.vi"("a phase"=w267, "reset"="Reset Encoder 5", "b phase"=w266, "z phase"=w265, "calls per sample"="calls per sample (vel)", "index criteria"=w261, "active states"=w260) -> ("encoder position"=w302:i32, "velocity"=w295:i16)  [unwired: 5 in, 2 out]
    n160 = Build Array(w306, w305, w304, w303, w302) -> (w301:i32[])
    n161 = Build Array(w299, w298, w297, w296, w295) -> (w300:i16[])
    n162 = global write "Global FPGA 5-axis.vi" "Unfiltered Position Feedback"(w301) -> ()
    n163 = global write "Global FPGA 5-axis.vi" "Unfiltered Velocity Feedback"(w300) -> ()
  }
  n164 = timed-loop "Synchronization Loop" {
    timing: w6 -> [_]
    timing-out: [_] -> w5
    stop <- FALSE stop-if-true
    n165 = xnode "FPGA I/O Node"() -> ("Scan Clock"=w322:bool)  [unwired: 1 in, 1 out]
    n166 = global read "Global FPGA 5-axis.vi" "Sync Enable"() -> (w321:bool)
    n167 = Select(t="Sync Value", s="Sync Enable override?", f=w321) -> (s? t:f=w318:bool)
    n168 = call-poly <vilib>:"nism.scan.generateSyncScan.vi"("scan enable?"=w318, "scan clock"=w322) -> ("timer control"=w323:T15)  [unwired: 3 in]
    n169 = global write "Global FPGA 5-axis.vi" "Timer Control"(w323) -> ()
  }
  n170 = timed-loop "Reset Monitoring Loop" {
    timing: w4 -> [_]
    timing-out: [_] -> w3
    stop <- FALSE stop-if-true
    n171 = global read "Global FPGA 5-axis.vi" "Reset Pending"() -> (w329:bool[])
    n172 = xnode "FPGA I/O Node"() -> ("Scan Clock"=w328:bool)  [unwired: 1 in, 1 out]
    n173 = feedback-in #1(w328) -> ()
    n174 = feedback #1() -> (w327:bool)  [unwired: 1 in]
    n175 = Greater?(x=w328, y=w327) -> (0:w333:bool)
    n176 = feedback #2() -> (w332:bool[])  [unwired: 1 in]
    n177 = Select(t=w329, s=w333, f=w332) -> (s? t:f=w330:bool[])
    n178 = feedback-in #2(w330) -> ()
    n179 = global write "Global FPGA 5-axis.vi" "Reset"(w330) -> ()
  }
  n180 = node-c288(w3) -> ()
  n181 = node-c288(w5) -> ()
  n182 = node-c288(w1) -> ()
  n183 = disable-structure shown="Disabled" {
    frame Disabled {
      # "Old code here, just in case."
      n184 = Index Array() -> (element #1=w346, element #2=w347, element #3=w348, element #4=w349, element #5=w350, element #6=w351)  [unwired: 7 in]
      n185 = shared-variable "NI-sbRIO9626-016FB69B\\User-Defined Variables\\Axis 1.Velocity Feedback"(w346) -> ()  [unwired: 1 in, 1 out]
      n186 = shared-variable "NI-sbRIO9626-016FB69B\\User-Defined Variables\\Axis 2.Velocity Feedback"(w347) -> ()  [unwired: 1 in, 1 out]
      n187 = shared-variable "NI-sbRIO9626-016FB69B\\User-Defined Variables\\Axis 3.Velocity Feedback"(w348) -> ()  [unwired: 1 in, 1 out]
      n188 = shared-variable "NI-sbRIO9626-016FB69B\\User-Defined Variables\\Axis 4.Velocity Feedback"(w349) -> ()  [unwired: 1 in, 1 out]
      n189 = shared-variable "NI-sbRIO9626-016FB69B\\User-Defined Variables\\Axis 5.Velocity Feedback"(w350) -> ()  [unwired: 1 in, 1 out]
      n190 = shared-variable "NI-sbRIO9626-016FB69B\\User-Defined Variables\\Axis 6.Velocity Feedback"(w351) -> ()  [unwired: 1 in, 1 out]
      n191 = Index Array() -> (element #1=w336, element #2=w337, element #3=w338, element #4=w339, element #5=w340, element #6=w341)  [unwired: 7 in]
      n192 = global read "Global FPGA 5-axis.vi" "Unfiltered Velocity Feedback"() -> (w344:i16[])
      n193 = shared-variable "NI-sbRIO9626-016FB69B\\User-Defined Variables\\Axis 1.Position Feedback"(w336) -> ()  [unwired: 1 in, 1 out]
      n194 = shared-variable "NI-sbRIO9626-016FB69B\\User-Defined Variables\\Axis 2.Position Feedback"(w337) -> ()  [unwired: 1 in, 1 out]
      n195 = shared-variable "NI-sbRIO9626-016FB69B\\User-Defined Variables\\Axis 3.Position Feedback"(w338) -> ()  [unwired: 1 in, 1 out]
      n196 = shared-variable "NI-sbRIO9626-016FB69B\\User-Defined Variables\\Axis 4.Position Feedback"(w339) -> ()  [unwired: 1 in, 1 out]
      n197 = shared-variable "NI-sbRIO9626-016FB69B\\User-Defined Variables\\Axis 5.Position Feedback"(w340) -> ()  [unwired: 1 in, 1 out]
      n198 = shared-variable "NI-sbRIO9626-016FB69B\\User-Defined Variables\\Axis 6.Position Feedback"(w341) -> ()  [unwired: 1 in, 1 out]
      n199 = Unbundle By Name("Encoder Config (Manual)") -> ("vel. filter coeffs."=w345:i32[])
      n200 = for {
        tunnel: "Velocity Filter Active?" -> [w355]
        tunnel: w345 -> [w354] mode=indexing
        tunnel: w344 -> [w353] mode=indexing
        tunnel: [w352] -> _ mode=indexing
        n201 = case shown="True" w355 {
          tunnel: w353 -> [w357 w361]
          tunnel: w354 -> [_ _]
          tunnel: [w356 w359] -> w352
          frame False {
            n202 = To Fixed-Point(number=w357) -> (fixed-point=w356:fxp<+/-,64,32>)  [unwired: 1 in]
          }
          frame True {
            n203 = To Fixed-Point(number=w361) -> (fixed-point=w360:fxp<+/-,16,16>)  [unwired: 1 in]
            n204 = xnode "Butterworth Filter"("input data"=w360) -> ("output data"=w358:fxp<+/-,16,16>)  [unwired: 2 in, 1 out]
            n205 = To Fixed-Point(number=w358) -> (fixed-point=w359:fxp<+/-,64,32>)  [unwired: 1 in]
          }
        }
      }
    }
    frame Enabled {
    }
  }
